vi "IR measure open.vi"(8 "error in (no error)":errorcluster) -> (0 "error out":errorcluster, 3 "ref array":refnum<class "IR sensor.lvclass">[](array[class]))   [LabVIEW 2019]
uses:
  FPGA_subVIs/low level/IR sensor/IR sensor.lvclass
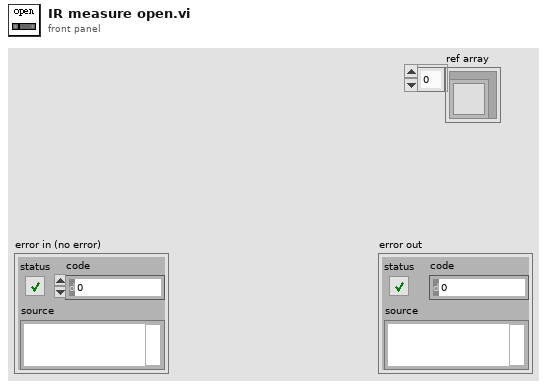
[diagram p1: front panel]
types:
  T1 = enum16{"IR.1", "IR.2", "IR.3", "IR.4", "IR.5", "IR.6", "IR.7", "IR.8"}
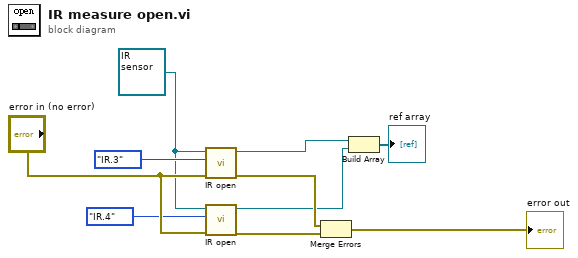
[diagram p0: block diagram]
diagram:
  w7 = refnum<class "IR sensor.lvclass"> refnum ("IR sensor in")
  n1 = call-dynamic "IR open.vi"("error in (no error)"="error in (no error)", "IR pin"=T1."IR.3", "IR sensor in"=w7) -> ("error out"=w6:errorcluster, "IR sensor out"=w3:refnum<class "IR sensor.lvclass">)  [unwired: 7 in]
  n2 = call-dynamic "IR open.vi"("error in (no error)"="error in (no error)", "IR pin"=T1."IR.4", "IR sensor in"=w7) -> ("error out"=w5:errorcluster, "IR sensor out"=w2:refnum<class "IR sensor.lvclass">)  [unwired: 7 in]
  n3 = Merge Errors(w6, w5) -> (→"error out":errorcluster)
  n4 = Build Array(w3, w2) -> (→"ref array":refnum<class "IR sensor.lvclass">[])
